vi "SNRDCOffsetStructure_ChangePowerFreq.vi"(8 "Analyze SNR Input":T1={"Pins"=["Xout"], "Published Data Id"=[], "frequency range"={"start frequency"=-1.0, "stop frequency"=-1.0}}, 9 "RFSG Input":T2={"LO configure setting"={"Carrier Frequency (Hz)"=5180000000.0, "Power Level(dBm)"=-10.0, "External Attenuation (dB)"=0.0}, "Port"=""} {"LO configure setting"."Carrier Frequency (Hz)" format="%#_6p"}, 10 "Scope Input":T3={"Min. Sample Rate"=1000000.0, "Min Record Length"=1000, "Vertical Coupling"=1, "Vertical Range (V)"=2.0, "Pins"=["Xout"]} {"Vertical Range (V)" format="%_3g"; "Vertical Coupling" items=["AC", "DC", "Ground"]; "Min. Sample Rate" format="%#_6p"}, 11 "Semiconductor Module Context":T4) -> (0 "error out":errorcluster)   [LabVIEW 2014]
uses:
  <vilib>/NI_TestStand_SemiconductorModule/NI_TestStand_Semiconductor_Module.lvlibp/PinMap/General/SemiconductorModuleContext.ctl
  Control/Scope Input.ctl
  Control/RFSG Input.ctl
  Control/Digitizier Analyze Input.ctl
  Control/Quene Type_Digitizer.ctl
  <vilib>/NI_TestStand_SemiconductorModule/NI_TestStand_Semiconductor_Module.lvlibp/PinMap/RF/RFPM/PinToNIRFPMSessions.vi
  <vilib>/NI_TestStand_SemiconductorModule/NI_TestStand_Semiconductor_Module.lvlibp
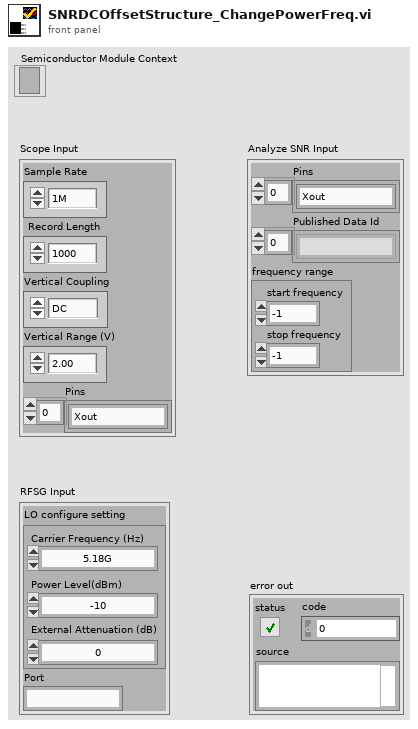
[diagram p1: front panel]
types:
  T1 = typedef "Digitizier Analyze Input.ctl" = cluster{"Pins":string[], "Published Data Id":string[], "frequency range":cluster{"start frequency":dbl, "stop frequency":dbl}}
  T2 = typedef "RFSG Input.ctl" = cluster{"LO configure setting":cluster{"Carrier Frequency (Hz)":dbl, "Power Level(dBm)":dbl, "External Attenuation (dB)":dbl}, "Port":string}
  T3 = typedef "Scope Input.ctl" = cluster{"Min. Sample Rate":dbl, "Min Record Length":i32, "Vertical Coupling":i32, "Vertical Range (V)":dbl, "Pins":string[]}
  T4 = typedef "NI_TestStand_Semiconductor_Module.lvlibp/SemiconductorModuleContext.ctl" = refnum<k7>
  T5 = typedef "Quene Type_Digitizer.ctl" = cluster{"Actiion":enum16{"Exit", "Analyze"}, "Waveform Data":waveform(dbl)[], "Semiconductor Module Context":T4, "error constant":errorcluster}
  T6 = cluster{"Carrier Frequency (Hz)":dbl, "Power Level(dBm)":dbl, "External Attenuation (dB)":dbl}
  T7 = cluster{"start frequency":dbl, "stop frequency":dbl}
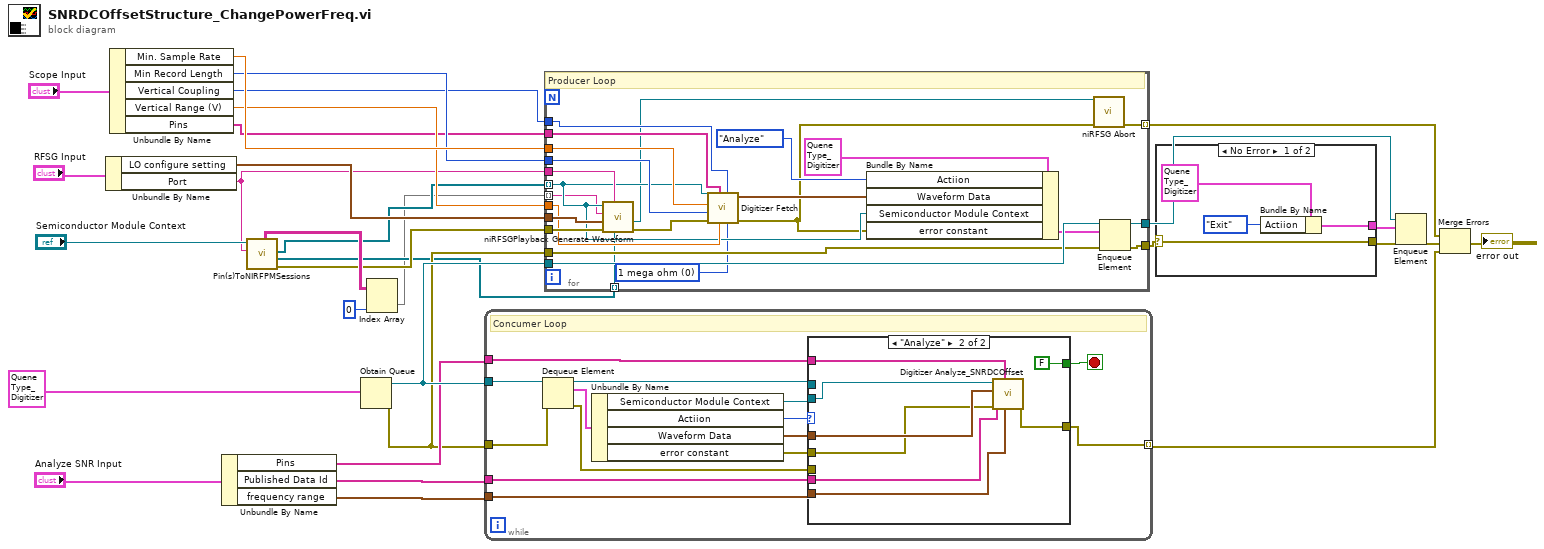
[diagram p0: block diagram]
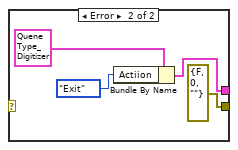
[diagram p2: hidden frame]
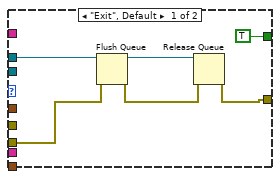
[diagram p3: hidden frame]
diagram:
  n1 = Unbundle By Name("RFSG Input") -> ("LO configure setting"=w29:T6, "Port"=w5:string)
  n2 = Unbundle By Name("Scope Input") -> ("Min. Sample Rate"=w27:dbl, "Min Record Length"=w26:i32, "Vertical Coupling"=w24:i32, "Vertical Range (V)"=w25:dbl, "Pins"=w23:string[])
  n3 = Unbundle By Name("Analyze SNR Input") -> ("Pins"=w17:string[], "Published Data Id"=w18:string[], "frequency range"=w19:T7)
  n4 = call-poly <vilib>:"Pin(s)ToNIRFPMSessions.vi"("Pin"=w5, "Semiconductor Module Context"="Semiconductor Module Context") -> ("error out"=w4:errorcluster, "Instrument Sessions"=w2:refnum<k15>[], "Semiconductor Module Contexts"=w3:refnum<k7>[], "Ports List"=w7:string[][])  [unwired: 4 in, 2 out]
  n5 = Obtain Queue(element data type=T5 {"Actiion"=enum."Analyze", "Waveform Data"=[], "Semiconductor Module Context"=refnum, "error constant"={"status"=FALSE, "code"=0, "source"=""}}) -> (queue out=w21:refnum<queue>, error out=w12:errorcluster)  [unwired: 4 in, 1 out]
  n6 = Index Array(array=w7, index (col)=0) -> (element=w1:string[])  [unwired: 1 in]
  n7 = while {
    tunnel: w21 -> [w45]
    tunnel: w19 -> [w39]
    tunnel: w18 -> [w38]
    tunnel: w17 -> [w37]
    tunnel: w12 -> [w44]
    tunnel: [w34] -> w14 mode=indexing
    stop <- w41 stop-if-true
    # "Concumer Loop"
    n8 = Dequeue Element(queue=w45, error in (no error)=w44) -> (queue out=w36:refnum<queue>, element=w43:T5, error out=w35:errorcluster)  [unwired: 1 in, 1 out]
    n9 = Unbundle By Name(w43) -> ("Semiconductor Module Context"=w33:T4, "Actiion"=w42:enum16{"Exit", "Analyze"}, "Waveform Data"=w40:waveform(dbl)[], "error constant"=w32:errorcluster)
    n10 = case shown="\"Analyze\"" w42 {
      tunnel: [TRUE FALSE] -> w41
      tunnel: w33 -> [_ w55]
      tunnel: w40 -> [_ w56]
      tunnel: w39 -> [_ w53]
      tunnel: w38 -> [_ w58]
      tunnel: w37 -> [_ w57]
      tunnel: w36 -> [w48 _]
      tunnel: w35 -> [w47 _]
      tunnel: [w46 w54] -> w34
      tunnel: w32 -> [_ w52]
      frame "Exit", Default {
        n11 = Flush Queue(queue=w48, error in (no error)=w47) -> (queue out=w50:refnum<queue>, error out=w49:errorcluster)  [unwired: 1 out]
        n12 = Release Queue(queue=w50, error in (no error)=w49) -> (error out=w46:errorcluster)  [unwired: 1 in, 2 out]
      }
      frame "Analyze" {
        n13 = call "Digitizer Analyze_SNRDCOffset.vi"("frequency range"=w53, "Pins"=w57, "error in"=w52, "Published Data Id"=w58, "Waveform Data In"=w56, "Semiconductor Module Context"=w55) -> ("error out"=w54:errorcluster)  [unwired: 2 in, 3 out]
      }
    }
  }
  n14 = for {
    tunnel: w3 -> [w66] mode=indexing
    tunnel: w29 -> [w82]
    tunnel: w5 -> [w81]
    tunnel: w27 -> [w80]
    tunnel: w26 -> [w79]
    tunnel: w25 -> [w77]
    tunnel: w24 -> [w76]
    tunnel: w23 -> [w75]
    tunnel: w21 -> [w74]
    tunnel: [w68] -> w22
    tunnel: w4 -> [w83]
    tunnel: [w65] -> w13 mode=indexing
    tunnel: w12 -> [w67]
    tunnel: [w69] -> w11
    tunnel: w2 -> [w63] mode=indexing
    tunnel: w1 -> [w62] mode=indexing
    w61 = u32 0 items=["1 mega ohm"=0, "50 ohms"=2] ("input impedance")
    # "Producer Loop"
    n15 = call "niRFSGPlayback Generate Waveform.vi"("instrument handle"=w63, "Port"=w81, "error in (no error)"=w83, "LO configure setting"=w82, "TX port"=w62, "TSM Context"=w66) -> ("error out"=w78:errorcluster, "instrument handle out"=w64:refnum<k15>)  [unwired: 4 in]
    n16 = call "Digitizer Fetch.vi"("input impedance"=w61, "Vertical Coupling"=w76, "Vertical Range (V)"=w77, "Pins"=w75, "error in (no error)"=w78, "Min Record Length"=w79, "Min. Sample Rate"=w80, "Semiconductor Module Context"=w66) -> ("error out"=w60:errorcluster, "Waveform Data Out"=w72:waveform(dbl)[])  [unwired: 2 in]
    n17 = Bundle By Name(cluster=T5 {"Actiion"=enum."Exit", "Waveform Data"=[], "Semiconductor Module Context"=refnum, "error constant"={"status"=FALSE, "code"=0, "source"=""}}, "Actiion"=enum16{"Exit", "Analyze"}."Analyze", "Waveform Data"=w72, "Semiconductor Module Context"=w66, "error constant"=w60) -> (w70:T5)
    n18 = call <instrlib>:"niRFSG Abort.vi"("instrument handle"=w64, "error in"=w60) -> ("error out"=w65:errorcluster)  [unwired: 12 in, 1 out]
    n19 = Enqueue Element(queue=w74, element=w70, error in (no error)=w67) -> (queue out=w68:refnum<queue>, error out=w69:errorcluster)  [unwired: 1 in, 1 out]
  }
  n20 = case shown="No Error" w11 {
    selector: w11 -> [w84 _]
    tunnel: [w85 w88] -> w10
    tunnel: [w84 errorcluster {"status"=FALSE, "code"=0, "source"=""} ("error IO")] -> w9
    frame No Error {
      n21 = Bundle By Name(cluster=T5 {"Actiion"=enum."Analyze", "Waveform Data"=[], "Semiconductor Module Context"=refnum, "error constant"={"status"=FALSE, "code"=0, "source"=""}}, "Actiion"=enum16{"Exit", "Analyze"}."Exit") -> (w85:T5)
    }
    frame Error {
      n22 = Bundle By Name(cluster=T5 {"Actiion"=enum."Analyze", "Waveform Data"=[], "Semiconductor Module Context"=refnum, "error constant"={"status"=FALSE, "code"=0, "source"=""}}, "Actiion"=enum16{"Exit", "Analyze"}."Exit") -> (w88:T5)
    }
  }
  n23 = Enqueue Element(queue=w22, element=w10, error in (no error)=w9) -> (error out=w15:errorcluster)  [unwired: 1 in, 2 out]
  n24 = Merge Errors(w13, w15, w14) -> (→"error out":errorcluster)
